vi "DataArray_SaveSelection.vi"(0 "Data Array":string[][](array[string]), 1 "SaveTemp":bool caption="Temperatures", 2 "SaveFreeze":bool caption="Freezing Point", 3 "SaveMelt":bool caption="Melting Point", 4 "SaveFrozen":bool caption="Frozen Fraction", 5 "Nm(T)":bool) -> (14 "Data Array out":string[][](array[string]))   [LabVIEW 2024]
panel:
  out "MainPart":string[][](array[string])
  out "Freeze Temps":string[][](array[string])
  out "Melt Temp":string[][](array[string])
  out "Frozen Fraction":string[][](array[string])
  out "TempArray":string[][](array[string])
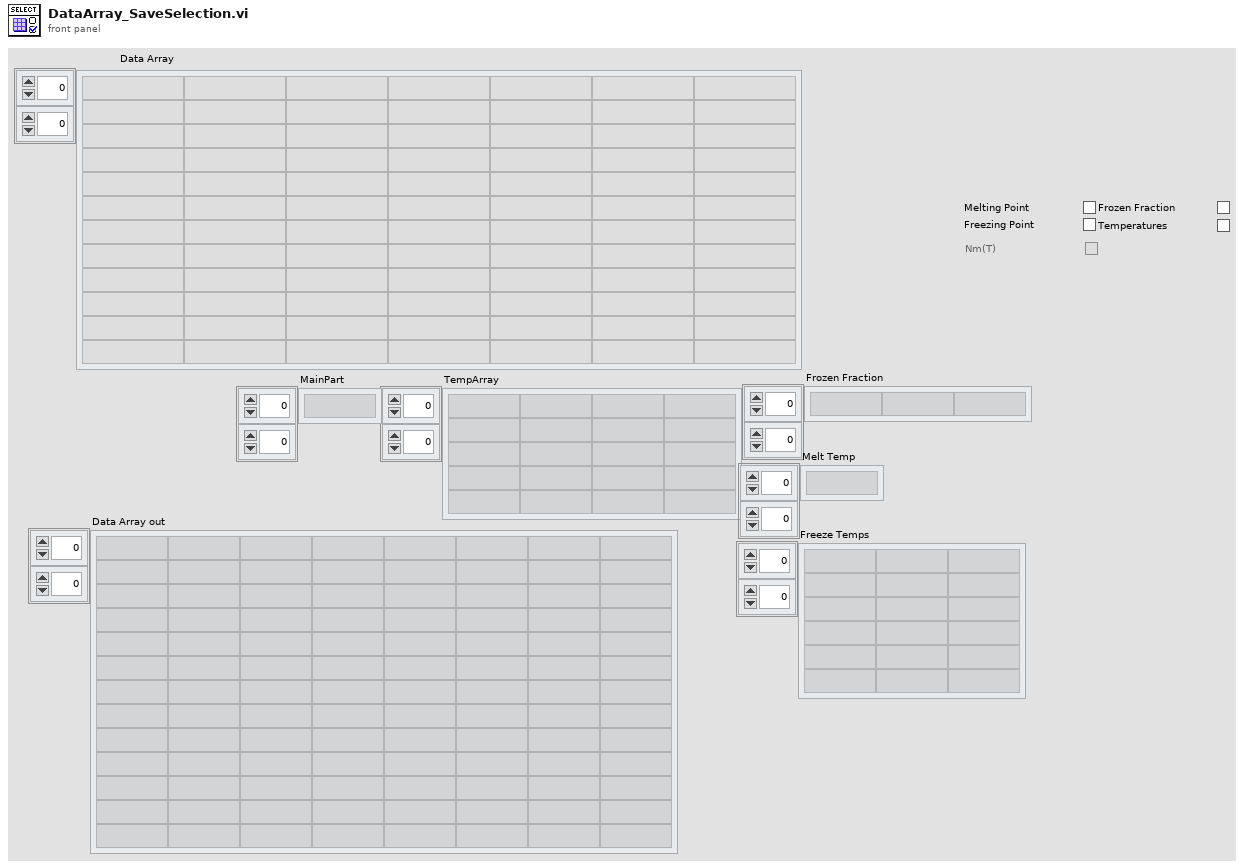
[diagram p1: front panel]
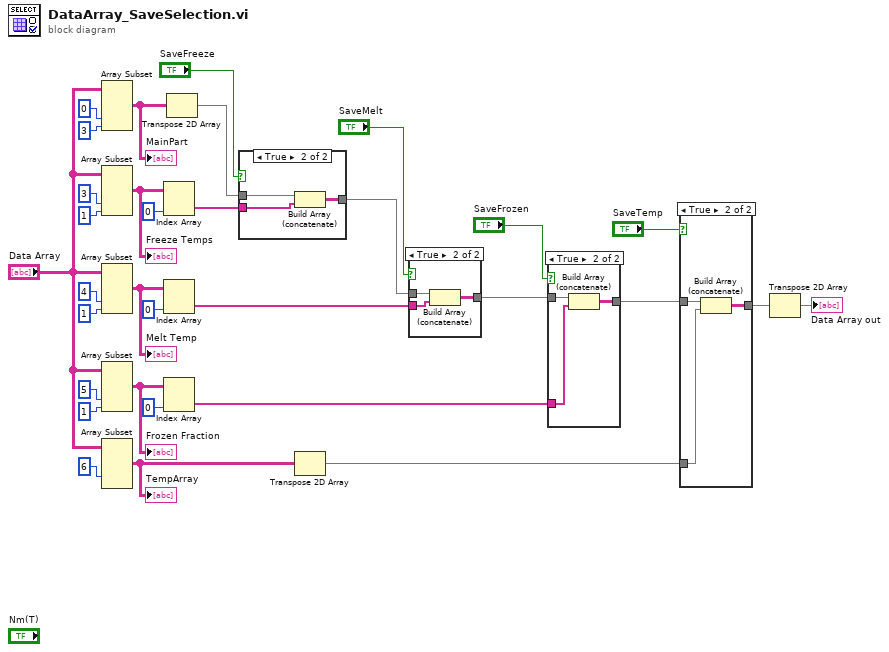
[diagram p0: block diagram]
diagram:
  n1 = Array Subset(array="Data Array", index (col)=0 ("index"), length (col)=3 ("length")) -> (w22:string[][])  [unwired: 2 in]
  "MainPart" <- w22
  n2 = Array Subset(array="Data Array", index (col)=3 ("index"), length (col)=1 ("length")) -> (w21:string[][])  [unwired: 2 in]
  "Freeze Temps" <- w21
  n3 = Array Subset(array="Data Array", index (col)=4 ("index"), length (col)=1 ("length")) -> (w20:string[][])  [unwired: 2 in]
  "Melt Temp" <- w20
  n4 = Array Subset(array="Data Array", index (col)=5 ("index"), length (col)=1 ("length")) -> (w19:string[][])  [unwired: 2 in]
  "Frozen Fraction" <- w19
  n5 = Array Subset(array="Data Array", index (col)=6 ("index")) -> (w18:string[][])  [unwired: 3 in]
  "TempArray" <- w18
  n6 = Index Array(array=w21, index (col)=0 ("disabled index (col)")) -> (element=w15:string[])  [unwired: 1 in]
  n7 = Index Array(array=w20, index (col)=0 ("disabled index (col)")) -> (element=w12:string[])  [unwired: 1 in]
  n8 = Index Array(array=w19, index (col)=0 ("disabled index (col)")) -> (element=w8:string[])  [unwired: 1 in]
  n9 = Transpose 2D Array(2D array=w22) -> (transposed array=w16:string[][])
  n10 = case shown="True" "SaveFreeze" {
    tunnel: w16 -> [w33 w36]
    tunnel: w15 -> [_ w35]
    tunnel: [w33 w34] -> w13
    frame False {
    }
    frame True {
      n11 = Build Array (concatenate)(w36, w35) -> (w34:string[][])
    }
  }
  n12 = Transpose 2D Array(2D array=w18) -> (transposed array=w5:string[][])
  n13 = case shown="True" "SaveMelt" {
    tunnel: w13 -> [w37 w40]
    tunnel: w12 -> [_ w39]
    tunnel: [w37 w38] -> w10
    frame False {
    }
    frame True {
      n14 = Build Array (concatenate)(w40, w39) -> (w38:string[][])
    }
  }
  n15 = case shown="True" "SaveFrozen" {
    tunnel: w10 -> [w41 w44]
    tunnel: w8 -> [_ w43]
    tunnel: [w41 w42] -> w7
    frame False {
    }
    frame True {
      n16 = Build Array (concatenate)(w44, w43) -> (w42:string[][])
    }
  }
  n17 = case shown="True" "SaveTemp" {
    tunnel: w7 -> [w45 w48]
    tunnel: w5 -> [_ w47]
    tunnel: [w45 w46] -> w4
    frame False {
    }
    frame True {
      n18 = Build Array (concatenate)(w48, w47) -> (w46:string[][])
    }
  }
  n19 = Transpose 2D Array(2D array=w4) -> (transposed array=→"Data Array out":string[][])
